vi "23_2.vi"() -> ()   [LabVIEW 2020]
uses:
  <vilib>/Analysis/1siggen.llb/Ramp Pattern by Delta.vi
  <vilib>/Analysis/NI_AALBase.lvlib
panel:
  out "Next Cup 2":i32
  out "Next Cup":i32
  out "Cup 1":i32
  in  "Moves":i32=100
  in  "Switch":bool
  in  "Input":string="925176834"
  in  "Input Test":string="389125467"
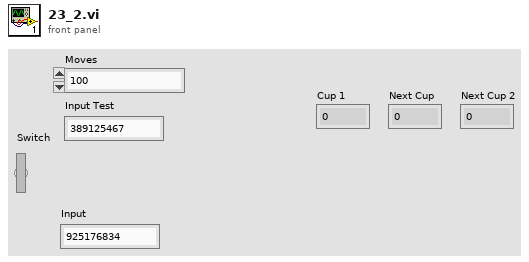
[diagram p1: front panel]
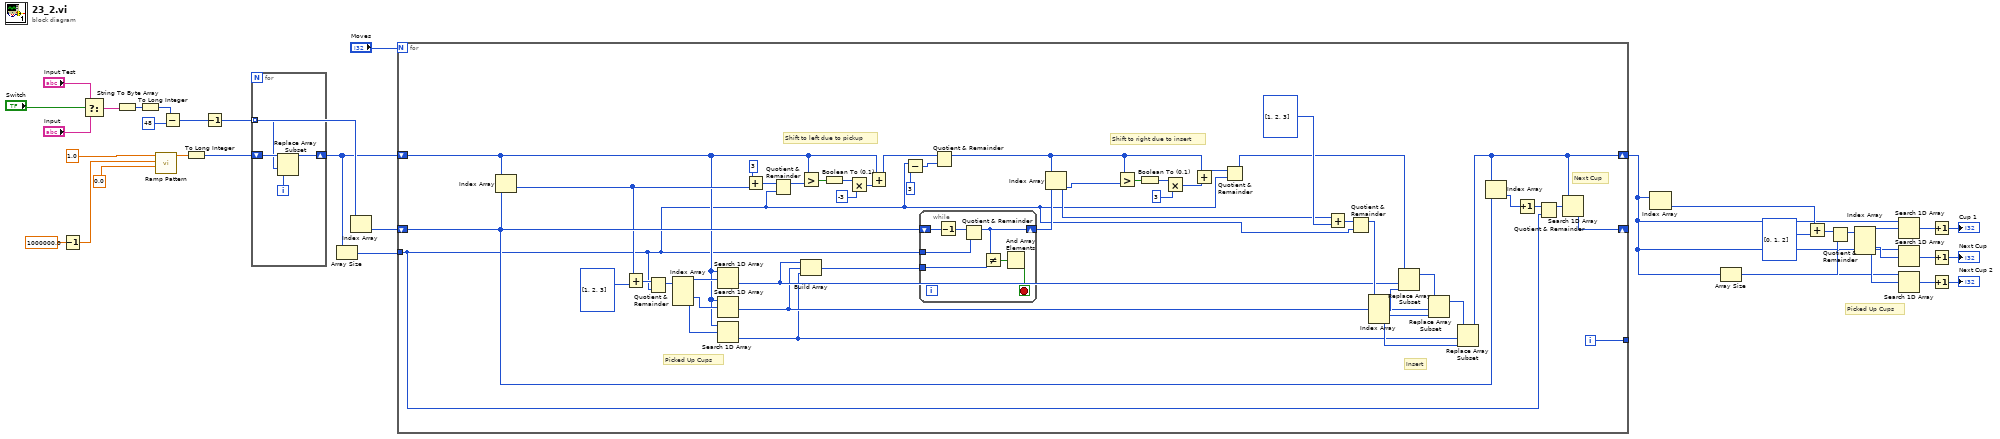
[diagram p0: block diagram]
diagram:
  # "Picked Up Cups"
  n1 = Decrement(x=1000000.0 ("end")) -> (x-1=w23:dbl)
  n2 = Select(t="Input Test", s="Switch", f="Input") -> (s? t:f=w31:string)
  n3 = String To Byte Array(string=w31) -> (unsigned byte array=w30:u8[])
  n4 = To Long Integer(number=w30) -> (32bit integer=w27:i32[])
  n5 = call-poly <vilib>:"Ramp Pattern.vi"("start"=0.0, "end"=w23, "delta"=1.0) -> ("Ramp Pattern"=w25:dbl[])  [unwired: 6 in, 2 out]
  n6 = Subtract(x=w27, y=48) -> (x-y=w22:i32[])
  n7 = To Long Integer(number=w25) -> (32bit integer=w18:i32[])
  n8 = Decrement(x=w22) -> (x-1=w20:i32[])
  n9 = for {
    tunnel: w20 -> [w36] mode=indexing
    shift-right: [w35] -> w17
    shift-left: w18 -> [w38]
    i -> [w37]
    n10 = Replace Array Subset(array=w38, new element=w37, index=w36) -> (w35:i32[])
  }
  n11 = Array Size(array=w17) -> (size(s)=w21:i32)
  n12 = Index Array(array=w20) -> (element=w19:i32)  [unwired: 1 in]
  n13 = for {
    N: "Moves" -> [_]
    shift-right: [w47] -> w1
    shift-left: w17 -> [w43]
    tunnel: [w85] -> _
    shift-right: [w50] -> _
    shift-left: w19 -> [w46]
    tunnel: w21 -> [w41]
    i -> [w85]
    # "Picked Up Cups"
    # "Next Cup"
    # "Insert"
    # "Shift to right due to insert"
    # "Shift to left due to pickup"
    n14 = Index Array(array=w43, index=w46) -> (element=w45:i32)
    n15 = Add(x=w45, y=i32[] [1, 2, 3]) -> (x+y=w72:i32[])
    n16 = Quotient & Remainder(x=w72, y=w41) -> (x-y*floor(x/y)=w71:i32[])  [unwired: 1 out]
    n17 = Index Array(array=w71) -> (element #1=w70:i32, element #2=w69:i32, element #3=w68:i32)  [unwired: 3 in]
    n18 = Search 1D Array(1D array=w43, element=w70) -> (index of element=w53:i32)  [unwired: 1 in]
    n19 = Search 1D Array(1D array=w43, element=w69) -> (index of element=w52:i32)  [unwired: 1 in]
    n20 = Search 1D Array(1D array=w43, element=w68) -> (index of element=w51:i32)  [unwired: 1 in]
    n21 = Add(x=3, y=w45) -> (x+y=w74:i32)
    n22 = Quotient & Remainder(x=w74, y=w41) -> (x-y*floor(x/y)=w59:i32)  [unwired: 1 out]
    n23 = Greater?(x=w43, y=w59) -> (0:w84:bool[])
    n24 = Build Array(w53, w52, w51) -> (w48:i32[])
    n25 = Boolean To (0,1)(Boolean=w84) -> (0, 1=w83:i16[])
    n26 = Multiply(x=w83, y=-3) -> (x*y=w81:i32[])
    n27 = Add(x=w43, y=w81) -> (x+y=w58:i32[])
    n28 = Subtract(x=w41, y=3) -> (x-y=w40:i32)
    n29 = while {
      tunnel: w41 -> [w90]
      shift-right: [w89] -> w49
      shift-left: w46 -> [w92]
      tunnel: w48 -> [w88]
      stop <- w86 stop-if-true
      n30 = Decrement(x=w92) -> (x-1=w91:i32)
      n31 = Quotient & Remainder(x=w91, y=w90) -> (x-y*floor(x/y)=w89:i32)  [unwired: 1 out]
      n32 = Not Equal?(x=w89, y=w88) -> (x != y?=w87:bool[])
      n33 = And Array Elements(Boolean array=w87) -> (logical AND=w86:bool)
    }
    n34 = Quotient & Remainder(x=w58, y=w40) -> (x-y*floor(x/y)=w55:i32[])  [unwired: 1 out]
    n35 = Index Array(array=w55, index=w49) -> (element=w42:i32)
    n36 = Greater?(x=w55, y=w42) -> (0:w77:bool[])
    n37 = Boolean To (0,1)(Boolean=w77) -> (0, 1=w78:i16[])
    n38 = Multiply(x=w78, y=3) -> (x*y=w80:i32[])
    n39 = Add(x=w55, y=w80) -> (x+y=w57:i32[])
    n40 = Quotient & Remainder(x=w57, y=w41) -> (x-y*floor(x/y)=w54:i32[])  [unwired: 1 out]
    n41 = Add(x=w42, y=i32[] [1, 2, 3]) -> (x+y=w65:i32[])
    n42 = Quotient & Remainder(x=w65, y=w41) -> (x-y*floor(x/y)=w63:i32[])  [unwired: 1 out]
    n43 = Index Array(array=w63) -> (element #1=w62:i32, element #2=w61:i32, element #3=w60:i32)  [unwired: 3 in]
    n44 = Replace Array Subset(array=w54, new element=w62, index=w53) -> (w67:i32[])
    n45 = Replace Array Subset(array=w67, new element=w61, index=w52) -> (w66:i32[])
    n46 = Replace Array Subset(array=w66, new element=w60, index=w51) -> (w47:i32[])
    n47 = Index Array(array=w47, index=w46) -> (element=w44:i32)
    n48 = Increment(x=w44) -> (x+1=w76:i32)
    n49 = Quotient & Remainder(x=w76, y=w41) -> (x-y*floor(x/y)=w75:i32)  [unwired: 1 out]
    n50 = Search 1D Array(1D array=w47, element=w75) -> (index of element=w50:i32)  [unwired: 1 in]
  }
  n51 = Index Array(array=w1) -> (element=w10:i32)  [unwired: 1 in]
  n52 = Array Size(array=w1) -> (size(s)=w6:i32)
  n53 = Add(x=w10, y=i32[] [0, 1, 2]) -> (x+y=w16:i32[])
  n54 = Quotient & Remainder(x=w16, y=w6) -> (x-y*floor(x/y)=w15:i32[])  [unwired: 1 out]
  n55 = Index Array(array=w15) -> (element #1=w14:i32, element #2=w13:i32, element #3=w12:i32)  [unwired: 3 in]
  n56 = Search 1D Array(1D array=w1, element=w14) -> (index of element=w9:i32)  [unwired: 1 in]
  n57 = Search 1D Array(1D array=w1, element=w13) -> (index of element=w8:i32)  [unwired: 1 in]
  n58 = Search 1D Array(1D array=w1, element=w12) -> (index of element=w7:i32)  [unwired: 1 in]
  n59 = Increment(x=w9) -> (x+1=→"Cup 1":i32)
  n60 = Increment(x=w8) -> (x+1=→"Next Cup":i32)
  n61 = Increment(x=w7) -> (x+1=→"Next Cup 2":i32)
